vi "Get Count LED Settings From Recipe.vi"(11 "Test Recipe in":refnum<class "Test Recipe.lvclass">) -> (0 "Minimum Artifact Size":dbl, 1 "Threshold Values":T1={"Red Range"={"Lower value"=0, "Upper value"=95}, "Green Range"={"Lower value"=0, "Upper value"=95}, "Blue Range"={"Lower value"=115, "Upper value"=255}}, 2 "Rectangle":T2 {"Rotation" format="%.2f"; "Left" scale=0.0..1024.0; "Right" scale=0.0..1024.0}, 3 "Search Settings":T3, 4 "Color?":bool, 5 "Exposure Speed":dbl, 6 "Save Image":bool)   [LabVIEW 2015, in "LED Board Test.lvclass"]
uses:
  LED Board Test.lvclass
  Classes/Test Recipe/Class/Test Recipe.lvclass
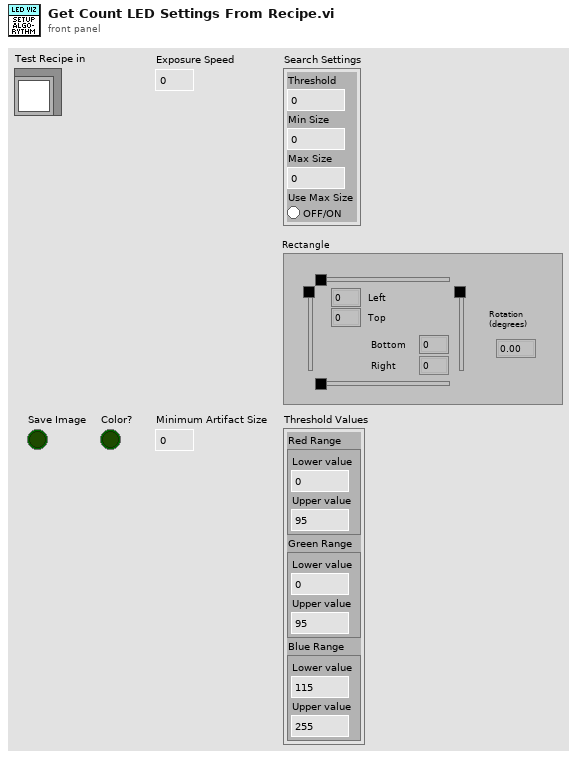
[diagram p1: front panel]
types:
  T1 = cluster{"Red Range":cluster{"Lower value":i32, "Upper value":i32}, "Green Range":cluster{"Lower value":i32, "Upper value":i32}, "Blue Range":cluster{"Lower value":i32, "Upper value":i32}}
  T2 = typedef "IMAQ Rectangle" = cluster{"Left":i32, "Top":i32, "Right":i32, "Bottom":i32, "Rotation":dbl}
  T3 = cluster{"Threshold":u32, "Min Size":u32, "Max Size":u32, "Use Max Size":bool}
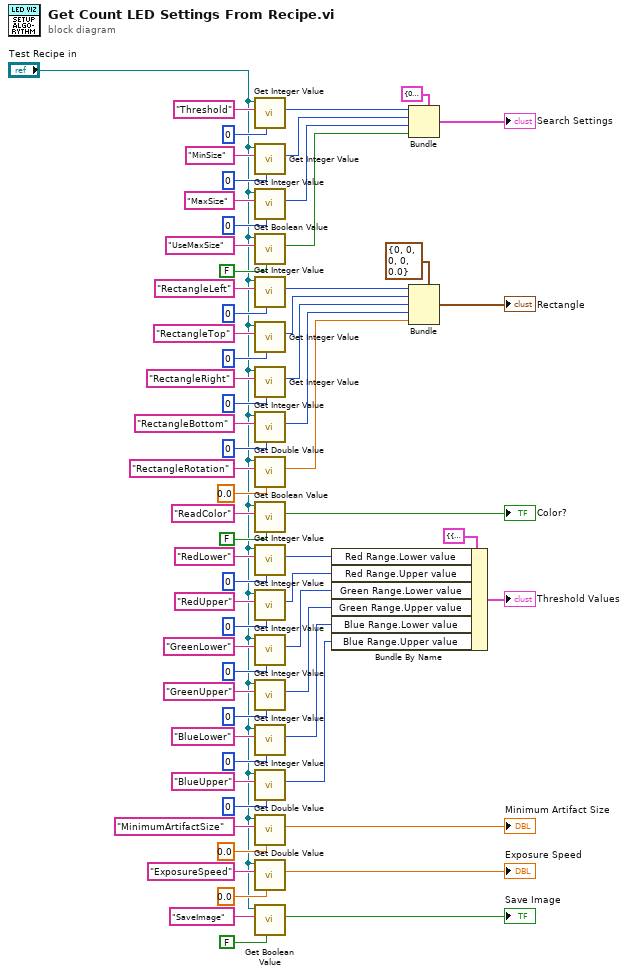
[diagram p0: block diagram]
diagram:
  n1 = call "Get Integer Value.vi"("Default Value"=u32 0, "Name"="Threshold", "Test Recipe in"="Test Recipe in") -> ("Value"=w54:i32)  [unwired: 5 in, 3 out]
  n2 = call "Get Integer Value.vi"("Default Value"=u32 0, "Name"="MinSize", "Test Recipe in"="Test Recipe in") -> ("Value"=w53:i32)  [unwired: 5 in, 3 out]
  n3 = call "Get Integer Value.vi"("Default Value"=u32 0, "Name"="MaxSize", "Test Recipe in"="Test Recipe in") -> ("Value"=w52:i32)  [unwired: 5 in, 3 out]
  n4 = call "Get Boolean Value.vi"("Default Value"=FALSE, "Name"="UseMaxSize", "Test Recipe in"="Test Recipe in") -> ("Value"=w51:bool)  [unwired: 5 in, 3 out]
  n5 = call "Get Integer Value.vi"("Default Value"=u32 0, "Name"="RectangleLeft", "Test Recipe in"="Test Recipe in") -> ("Value"=w38:i32)  [unwired: 5 in, 3 out]
  n6 = call "Get Integer Value.vi"("Default Value"=u32 0, "Name"="RectangleTop", "Test Recipe in"="Test Recipe in") -> ("Value"=w37:i32)  [unwired: 5 in, 3 out]
  n7 = call "Get Integer Value.vi"("Default Value"=u32 0, "Name"="RectangleRight", "Test Recipe in"="Test Recipe in") -> ("Value"=w36:i32)  [unwired: 5 in, 3 out]
  n8 = call "Get Integer Value.vi"("Default Value"=u32 0, "Name"="RectangleBottom", "Test Recipe in"="Test Recipe in") -> ("Value"=w35:i32)  [unwired: 5 in, 3 out]
  n9 = call "Get Double Value.vi"("Default Value"=0.0, "Name"="RectangleRotation", "Test Recipe in"="Test Recipe in") -> ("Value"=w32:dbl)  [unwired: 5 in, 3 out]
  n10 = call "Get Boolean Value.vi"("Default Value"=FALSE, "Name"="ReadColor", "Test Recipe in"="Test Recipe in") -> ("Value"=→"Color?":bool)  [unwired: 5 in, 3 out]
  n11 = call "Get Integer Value.vi"("Default Value"=u32 0, "Name"="RedLower", "Test Recipe in"="Test Recipe in") -> ("Value"=w17:i32)  [unwired: 5 in, 3 out]
  n12 = call "Get Integer Value.vi"("Default Value"=u32 0, "Name"="RedUpper", "Test Recipe in"="Test Recipe in") -> ("Value"=w16:i32)  [unwired: 5 in, 3 out]
  n13 = call "Get Integer Value.vi"("Default Value"=u32 0, "Name"="GreenLower", "Test Recipe in"="Test Recipe in") -> ("Value"=w15:i32)  [unwired: 5 in, 3 out]
  n14 = call "Get Integer Value.vi"("Default Value"=u32 0, "Name"="GreenUpper", "Test Recipe in"="Test Recipe in") -> ("Value"=w14:i32)  [unwired: 5 in, 3 out]
  n15 = call "Get Integer Value.vi"("Default Value"=u32 0, "Name"="BlueLower", "Test Recipe in"="Test Recipe in") -> ("Value"=w13:i32)  [unwired: 5 in, 3 out]
  n16 = call "Get Integer Value.vi"("Default Value"=u32 0, "Name"="BlueUpper", "Test Recipe in"="Test Recipe in") -> ("Value"=w12:i32)  [unwired: 5 in, 3 out]
  n17 = call "Get Double Value.vi"("Default Value"=0.0, "Name"="MinimumArtifactSize", "Test Recipe in"="Test Recipe in") -> ("Value"=→"Minimum Artifact Size":dbl)  [unwired: 5 in, 3 out]
  n18 = call "Get Double Value.vi"("Default Value"=0.0, "Name"="ExposureSpeed", "Test Recipe in"="Test Recipe in") -> ("Value"=→"Exposure Speed":dbl)  [unwired: 5 in, 3 out]
  n19 = call "Get Boolean Value.vi"("Default Value"=FALSE, "Name"="SaveImage", "Test Recipe in"="Test Recipe in") -> ("Value"=→"Save Image":bool)  [unwired: 5 in, 3 out]
  n20 = Bundle By Name(cluster=T1 {"Red Range"={"Lower value"=0, "Upper value"=95}, "Green Range"={"Lower value"=0, "Upper value"=95}, "Blue Range"={"Lower value"=115, "Upper value"=255}} ("Threshold Values"), "Red Range.Lower value"=w17, "Red Range.Upper value"=w16, "Green Range.Lower value"=w15, "Green Range.Upper value"=w14, "Blue Range.Lower value"=w13, "Blue Range.Upper value"=w12) -> (→"Threshold Values":T1)
  n21 = Bundle(cluster=T3 {"Threshold"=0, "Min Size"=0, "Max Size"=0, "Use Max Size"=FALSE}, "Threshold"=w54, "Min Size"=w53, "Max Size"=w52, "Use Max Size"=w51) -> (→"Search Settings":T3)
  n22 = Bundle(cluster=T2 {"Left"=0, "Top"=0, "Right"=0, "Bottom"=0, "Rotation"=0.0} ("Rectangle"), "Left"=w38, "Top"=w37, "Right"=w36, "Bottom"=w35, "Rotation"=w32) -> (→"Rectangle":T2)
